vi "Channel 3  Adc Conversion.vi"(8 "Error In":errorcluster, 11 "Adc Convertor In":refnum<class "Adc Convertor.lvclass">) -> (0 "Error Out":errorcluster, 3 "Adc Convertor Out":refnum<class "Adc Convertor.lvclass">)   [LabVIEW 2021, in "Adc Convertor.lvclass"]
doc: "This VI converts the analog data to digital data of channel 3"
uses:
  Adc Convertor.lvclass
  <vilib>/numeric/Random Number (Range) DBL.vi
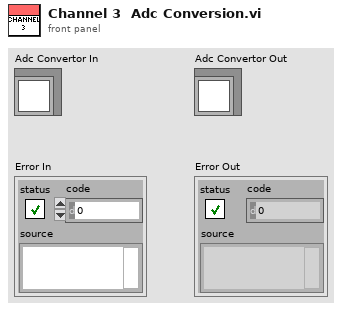
[diagram p1: front panel]
types:
  T1 = typedef "Channel Data.ctl" = cluster{"Channel 1 U8  Array":u8[], "Channel 2 U8  Array ":u8[], "Channel 3 U8  Array":u8[], "Channel 4 U8  Array":u8[]}
  T2 = typedef "ADC Type.ctl" = cluster{"Channels":string, "Range":dbl, "Resolution":dbl, "Sampling Rate":dbl}
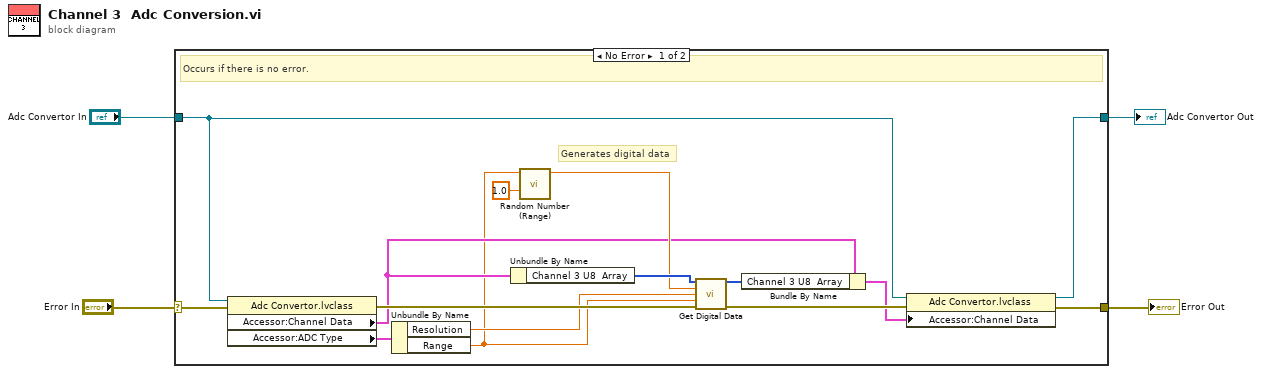
[diagram p0: block diagram]
diagram:
  n1 = case shown="No Error" "Error In" {
    selector: "Error In" -> [w10 w21]
    tunnel: [w9 w21] -> w3
    tunnel: [w7 w20] -> w1
    tunnel: "Adc Convertor In" -> [w8 w20]
    frame No Error {
      # "Generates digital data"
      # "Occurs if there is no error."
      n2 = property class="Adc Convertor.lvclass"(reference=w8, error in=w10) -> (error out=w18:errorcluster, "Accessor:Channel Data"=w6:T1, "Accessor:ADC Type"=w16:T2)  [unwired: 1 out]
      n3 = Unbundle By Name(w16) -> ("Resolution"=w15:dbl, "Range"=w5:dbl)
      n4 = Unbundle By Name(w6) -> ("Channel 3 U8  Array"=w17:u8[])
      n5 = call-poly <vilib>:"Random Number (Range).vi"("lower bound (0)"=1.0, "upper bound (100)"=w5) -> ("number"=w11:dbl)  [unwired: 9 in]
      n6 = call "Get Digital Data.vi"("Input Array"=w17, "Analog Input"=w11, "Resolution"=w15, "Range"=w5, "Error In"=w18) -> ("Output Array"=w14:u8[], "Error Out"=w19:errorcluster)  [unwired: 9 in]
      n7 = Bundle By Name(cluster=w6, "Channel 3 U8  Array"=w14) -> (w13:T1)
      n8 = property class="Adc Convertor.lvclass"(reference=w8, error in=w19, "Accessor:Channel Data"=w13) -> (reference out=w7:refnum<class "Adc Convertor.lvclass">, error out=w9:errorcluster)
    }
    frame Error {
      # "Occurs if there is any error."
    }
  }
  "Error Out" <- w3
  "Adc Convertor Out" <- w1
